vi "Add User.vi"(8 "error in (no error)":errorcluster, 10 "Credential":T1, 11 "Access in":refnum<class "Access.lvclass">) -> (0 "error out":errorcluster, 3 "Access out":refnum<class "Access.lvclass">)   [LabVIEW 2016, in "Database.lvlib" / "Access.lvclass"]
uses:
  Access.lvclass
  DB/Credential.ctl
  <vilib>/addons/database/NI_Database_API.lvlib
  User Interface/User Interface.lvlib
  Database.lvlib
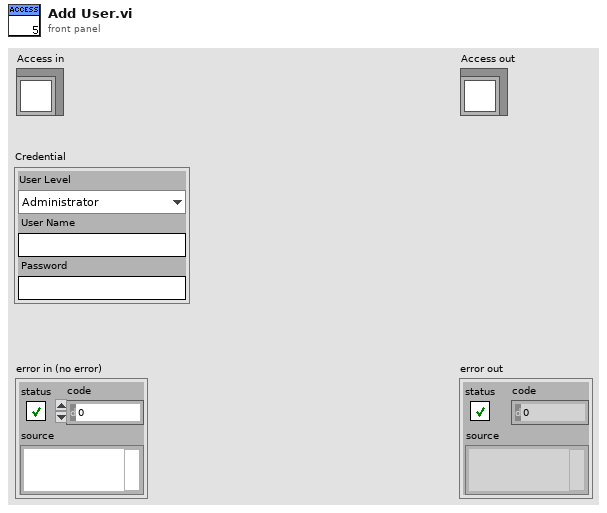
[diagram p1: front panel]
types:
  T1 = typedef "Database.lvlib/Credential.ctl" = cluster{"User Level":enum16{"Administrator", "Engineer", "Operator"}, "User Name":string, "Password":string}
  T2 = typedef "Database.lvlib/DB.lvclass/Table_info.ctl" = cluster{"Authentication":string, "Instr_Configuration":string, "Recipe":string, "Test_data":string}
  T3 = typedef "NI_Database_API.lvlib/Conn ObjectReference.ctl" = refnum<k1>
  T4 = cluster{"date/time string":string, string, "User Name":string, "Password":string}
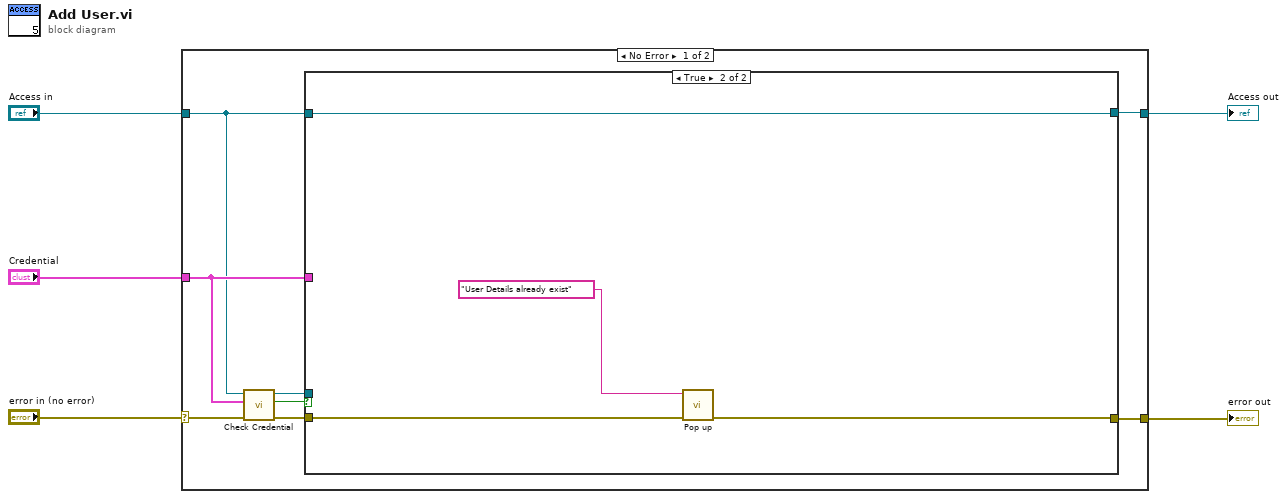
[diagram p0: block diagram]
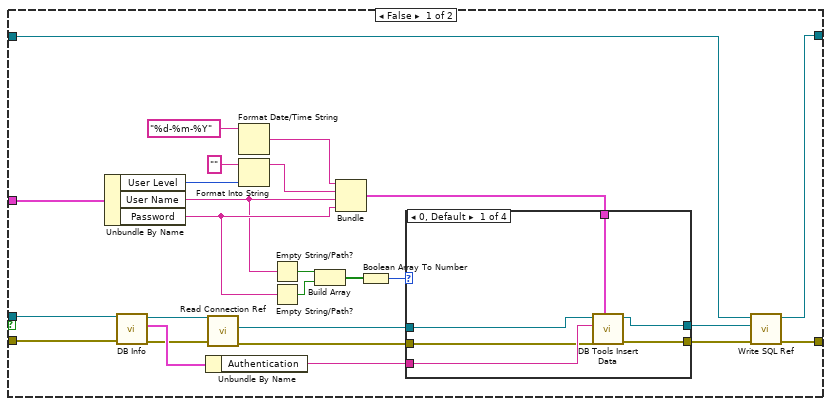
[diagram p2: hidden frame]
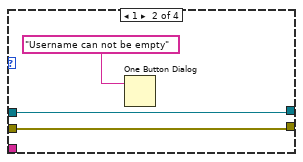
[diagram p3: hidden frame]
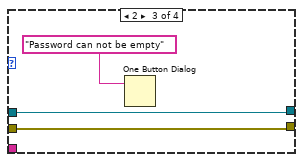
[diagram p4: hidden frame]
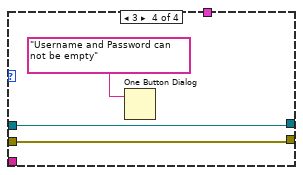
[diagram p5: hidden frame]
diagram:
  n1 = case shown="No Error" "error in (no error)" {
    selector: "error in (no error)" -> [w13 w59]
    tunnel: [w7 w60] -> w4
    tunnel: "Access in" -> [w8 w60]
    tunnel: [w6 w59] -> w2
    tunnel: "Credential" -> [w12 _]
    frame No Error {
      n2 = call-dynamic "Check Credential.vi"("error in (no error)"=w13, "Credential"=w12, "Access in"=w8) -> ("error out"=w10:errorcluster, "Match?"=w9:bool, "Access out"=w11:refnum<class "Access.lvclass">)  [unwired: 6 in]
      n3 = case shown="True" w9 {
        tunnel: [w16 w55] -> w6
        tunnel: w12 -> [w23 _]
        tunnel: w11 -> [w22 _]
        tunnel: w10 -> [w21 w57]
        tunnel: w8 -> [w18 w58]
        tunnel: [w17 w58] -> w7
        frame False {
          n4 = Unbundle By Name(w23) -> ("User Level"=w37:enum16{"Administrator", "Engineer", "Operator"}, "User Name"=w28:string, "Password"=w29:string)
          n5 = call-dynamic "DB Info.vi"("error in (no error)"=w21, "Access in"=w22) -> ("error out"=w33:errorcluster, "Table_info"=w39:T2, "Access out"=w32:refnum<class "Access.lvclass">)  [unwired: 6 in, 1 out]
          n6 = Unbundle By Name(w39) -> ("Authentication"=w38:string)
          n7 = call-dynamic "Read Connection Ref.vi"("error in (no error)"=w33, "Access in"=w32) -> ("error out"=w31:errorcluster, "connection reference"=w30:T3)  [unwired: 7 in, 1 out]
          n8 = Format Date/Time String(time format string (%c)="%d-%m-%Y") -> (date/time string=w14:string)  [unwired: 2 in]
          n9 = Format Into String(initial string="", w37) -> (resulting string=w35:string)  [unwired: 2 in, 1 out]
          n10 = Empty String/Path?(string/path=w28) -> (empty?=w27:bool)
          n11 = Empty String/Path?(string/path=w29) -> (empty?=w26:bool)
          n12 = Build Array(w27, w26) -> (w25:bool[])
          n13 = Bundle("date/time string"=w14, w35, "User Name"=w28, "Password"=w29) -> (w34:T4)  [unwired: 1 in]
          n14 = Boolean Array To Number(Boolean array=w25) -> (number=w24:u32)
          n15 = case shown="0, Default" w24 {
            tunnel: [w45 w46 w49 w52] -> w20
            tunnel: w38 -> [w44 _ _ _]
            tunnel: [w43 w47 w50 w53] -> w19
            tunnel: w34 -> [w42 _ _ _]
            tunnel: w31 -> [w41 w46 w49 w52]
            tunnel: w30 -> [w40 w47 w50 w53]
            frame 0, Default {
              n16 = call <vilib>:"DB Tools Insert Data.vi"("data"=w42, "error in (no error)"=w41, "table"=w44, "connection reference"=w40) -> ("error out"=w45:errorcluster, "connection reference out"=w43:T3)  [unwired: 6 in]
            }
            frame 1 {
              n17 = One Button Dialog(message="Username can not be empty") -> ()  [unwired: 1 in, 1 out]
            }
            frame 2 {
              n18 = One Button Dialog(message="Password can not be empty") -> ()  [unwired: 1 in, 1 out]
            }
            frame 3 {
              n19 = One Button Dialog(message="Username and Password can not be empty") -> ()  [unwired: 1 in, 1 out]
            }
          }
          n20 = call-dynamic "Write SQL Ref.vi"("error in (no error)"=w20, "connection reference"=w19, "Access in"=w18) -> ("error out"=w16:errorcluster, "Access out"=w17:refnum<class "Access.lvclass">)  [unwired: 7 in]
        }
        frame True {
          n21 = call "Pop up.vi"("error in (no error)"=w57, "Message In"="User Details already exist" ("message")) -> ("error out"=w55:errorcluster)  [unwired: 9 in]
        }
      }
    }
    frame Error {
    }
  }
  "error out" <- w2
  "Access out" <- w4
